vi "Check Loop Error.vi"(9 "Ignore Errors":i32[](array[numeric]) caption="에러 무시", 10 "error to process":errorcluster caption="처리할 에러", 11 "Message Queue":refnum<queue> caption="메시지 큐") -> (2 "Enqueued Error?":bool caption="큐에 추가된 에러?", 3 "dup Message Queue":refnum<queue> caption="메시지 큐 복제")   [LabVIEW 2018, in "Message Queue.lvlib"]
doc: "'처리할 에러'의 코드값이 '에러 무시' 배열의 값과 하나라도 일치하는지 확인합니다. 일치하는 경우, 아무 작업도 하지 않습니다. 일치하지 않는 경우, 에러 데이터를 포함하는 \"에러\" 메시지를 메시지 핸들링 루프로 보내 처리되도록 합니다."
uses:
  Message Queue.lvlib
  Enqueue Message (Single).vi
  Message Cluster.ctl
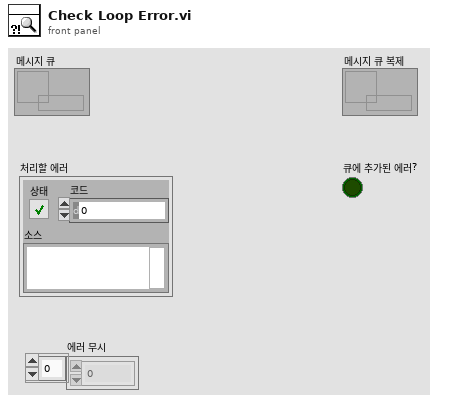
[diagram p1: front panel]
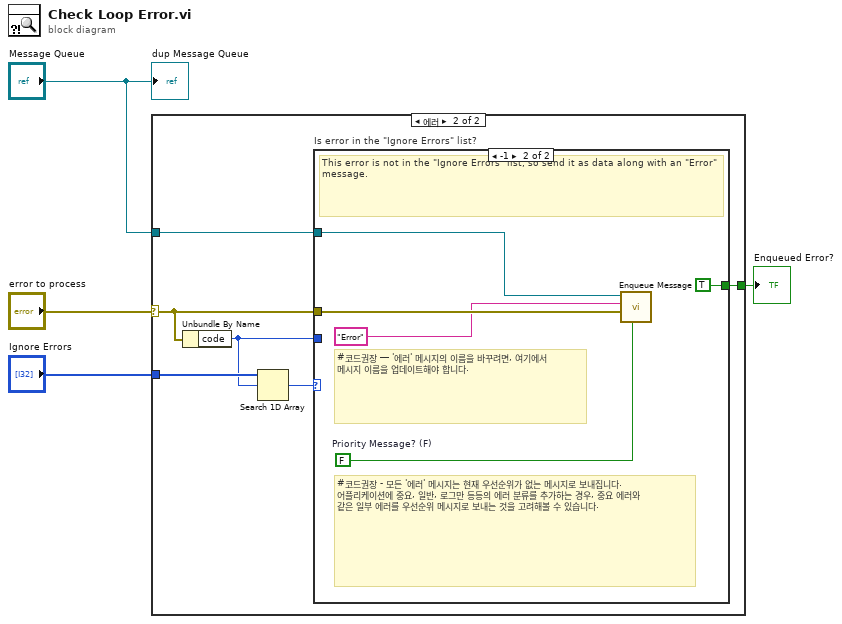
[diagram p0: block diagram]
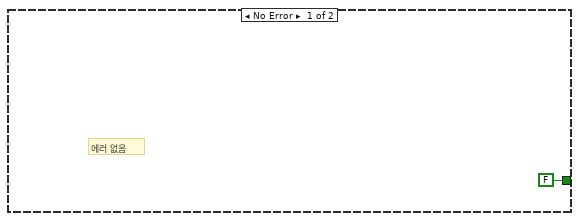
[diagram p2: hidden frame]
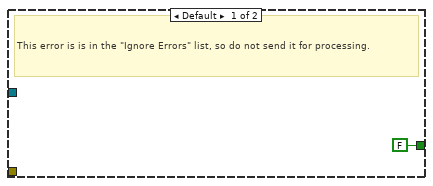
[diagram p3: hidden frame]
diagram:
  n1 = case shown="에러" "error to process" {
    selector: "error to process" -> [_ w7]
    tunnel: "Ignore Errors" -> [_ w11]
    tunnel: "Message Queue" -> [_ w9]
    tunnel: [FALSE ("Enqueued Error?") w6] -> w1
    frame No Error {
      # "에러 없음"
    }
    frame Error {
      n2 = Unbundle By Name(w7) -> ("code"=w8:i32)
      n3 = Search 1D Array(1D array=w11, element=w8) -> (index of element=w10:i32)  [unwired: 1 in]
      n4 = case "Is error in the \"Ignore Errors\" list?" shown="-1" w10 {
        tunnel: w9 -> [_ w16]
        tunnel: w8 -> [_ _]
        tunnel: w7 -> [_ w17]
        tunnel: [FALSE ("Enqueued Error?") TRUE ("Enqueued Error?")] -> w6
        frame Default {
          # "This error is is in the \"Ignore Errors\" list, so do not send it for processing."
        }
        frame -1 {
          w14 = FALSE  # Priority Message? (F)
          # "#코드권장 - 모든 '에러' 메시지는 현재 우선순위가 없는 메시지로 보내집니다. 어플리케이션에 중요, 일반, 로그만 등등의 에러 분류를 추가하는 경우, 중요 에러와 같은 일부 에러를 우선순위 메시지로 보내는 것을 고려해볼 수 있습니다."
          # "#코드권장 ― '에러' 메시지의 이름을 바꾸려면, 여기에서 메시지 이름을 업데이트해야 합니다."
          # "This error is not in the \"Ignore Errors\" list, so send it as data along with an \"Error\" message."
          n5 = call-poly "Enqueue Message.vi"("Priority Message? (F)"=w14, "Message Data"=w17, "Message"="Error", "Message Queue"=w16) -> ()  [unwired: 6 in, 2 out]
        }
      }
    }
  }
  "Enqueued Error?" <- w1
  "dup Message Queue" <- "Message Queue"
